vi "demo 0.vi"() -> ()   [LabVIEW 2023]
uses:
  <vilib>/addons/database/Auxilliary.llb/DB Tools Column Info.ctl
  <vilib>/addons/database/Auxilliary.llb/DB Tools DataTypes.ctl
  <vilib>/addons/database/Connection.llb/DB Tools Open Connec (Path).vi
  <vilib>/addons/database/_DB Variant To Data/Database Variant To Data.xnode
  <vilib>/addons/database/NI_Database_API.lvlib
panel:
  in  "?":bool
  out "Attention":string="TYPES YOUR INFORMATIONS "
  in  "connection information 3":path
  in  "column information":T1[](array[typedef])=[{"column name"="stringcol", "data type"=enum."String", "size"=50, "allow null?"=FALSE}, {"column name"="intcol", "data type"=enum."Long (I32)", "size"=0, "allow null?"=TRUE}, {"column name"="doublecol", "data type"=enum."Double (DBL)", "size"=0, "allow null?"=TRUE}]
  in  "LOGING":T3={"PRENOM"="This is a test string", "NOM"="This is a test string", "  TEL"="This is a test string"}
  in  "connection information":path
  out "?":string[][](array[string])
  out "error out":errorcluster
  # "NOM"
  # "TEL"
  # "PRENOM"
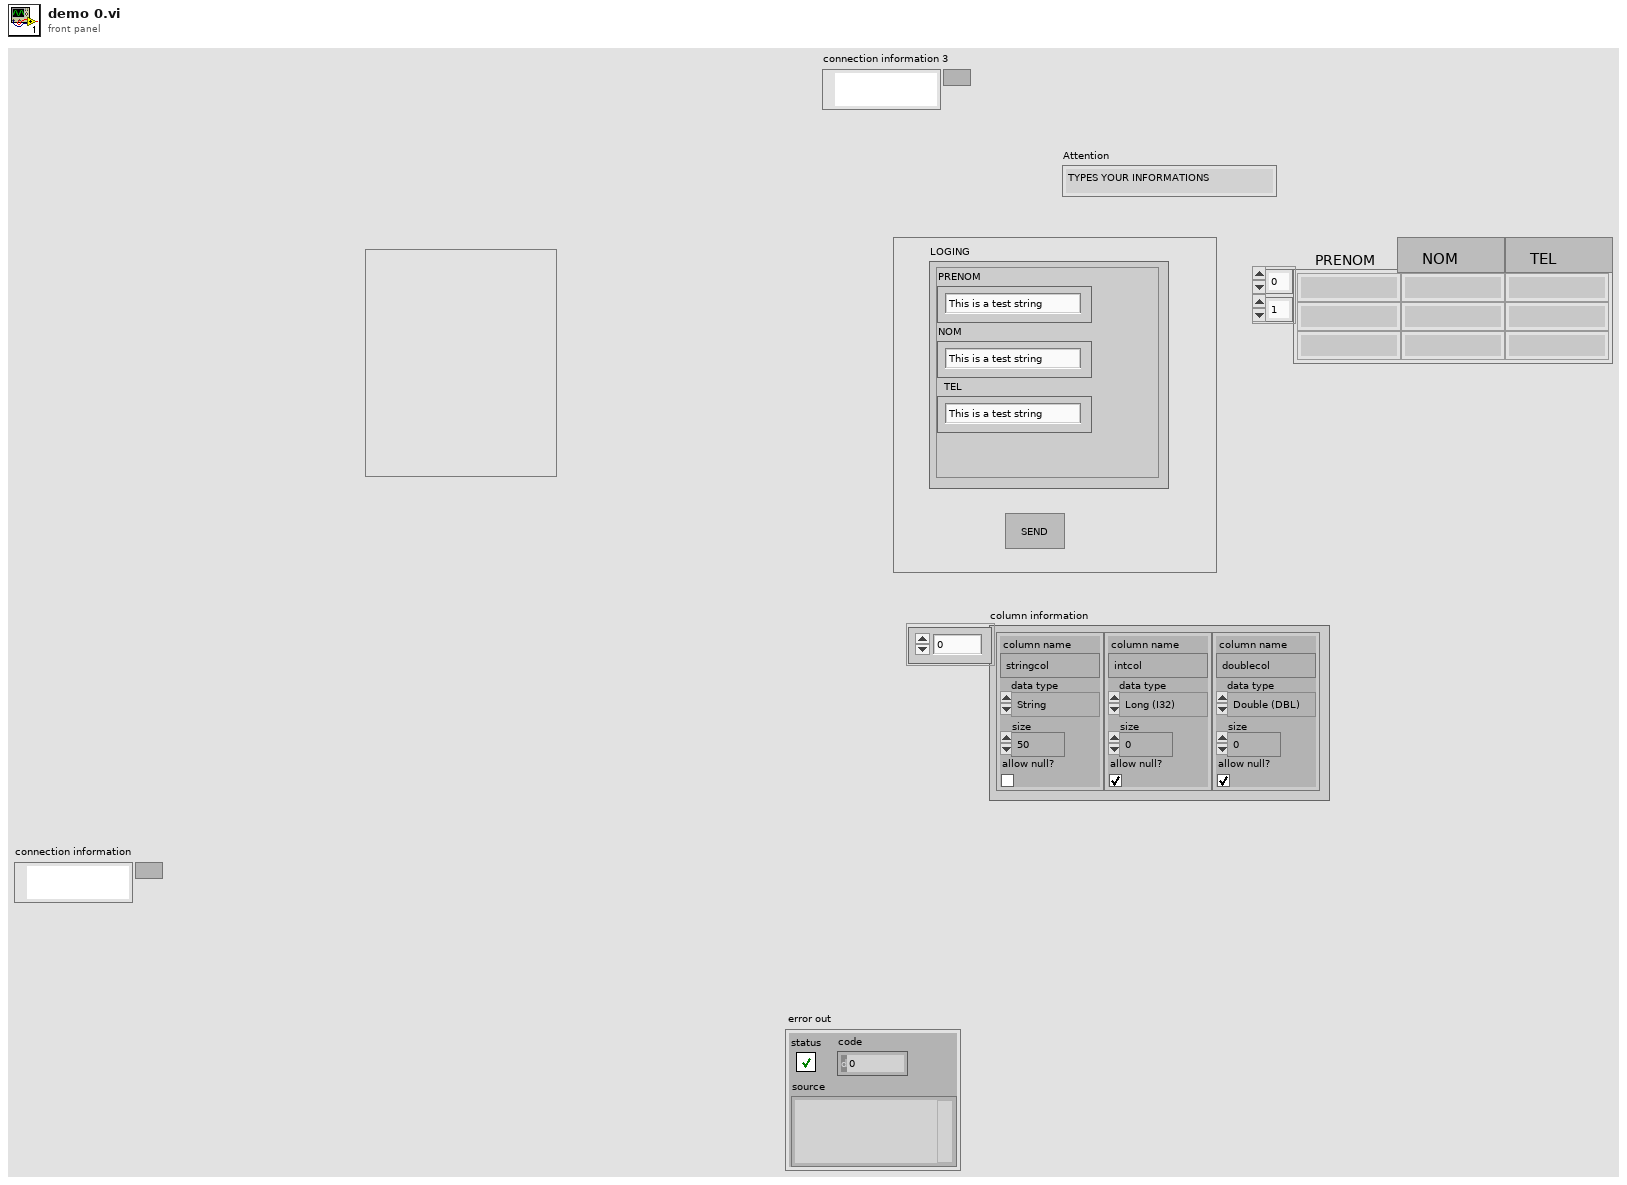
[diagram p1: front panel]
types:
  T1 = typedef "NI_Database_API.lvlib/DB Tools Column Info.ctl" = cluster{"column name":string, "data type":T2, "size":i32, "allow null?":bool}
  T2 = typedef "NI_Database_API.lvlib/DB Tools DataTypes.ctl" = enum16{"String", "Long (I32)", "Single (SGL)", "Double (DBL)", "Date/Time", "Binary"}
  T3 = cluster{"PRENOM":string, "NOM":string, "  TEL":string}
  T4 = typedef "NI_Database_API.lvlib/Conn ObjectReference.ctl" = refnum<k1>
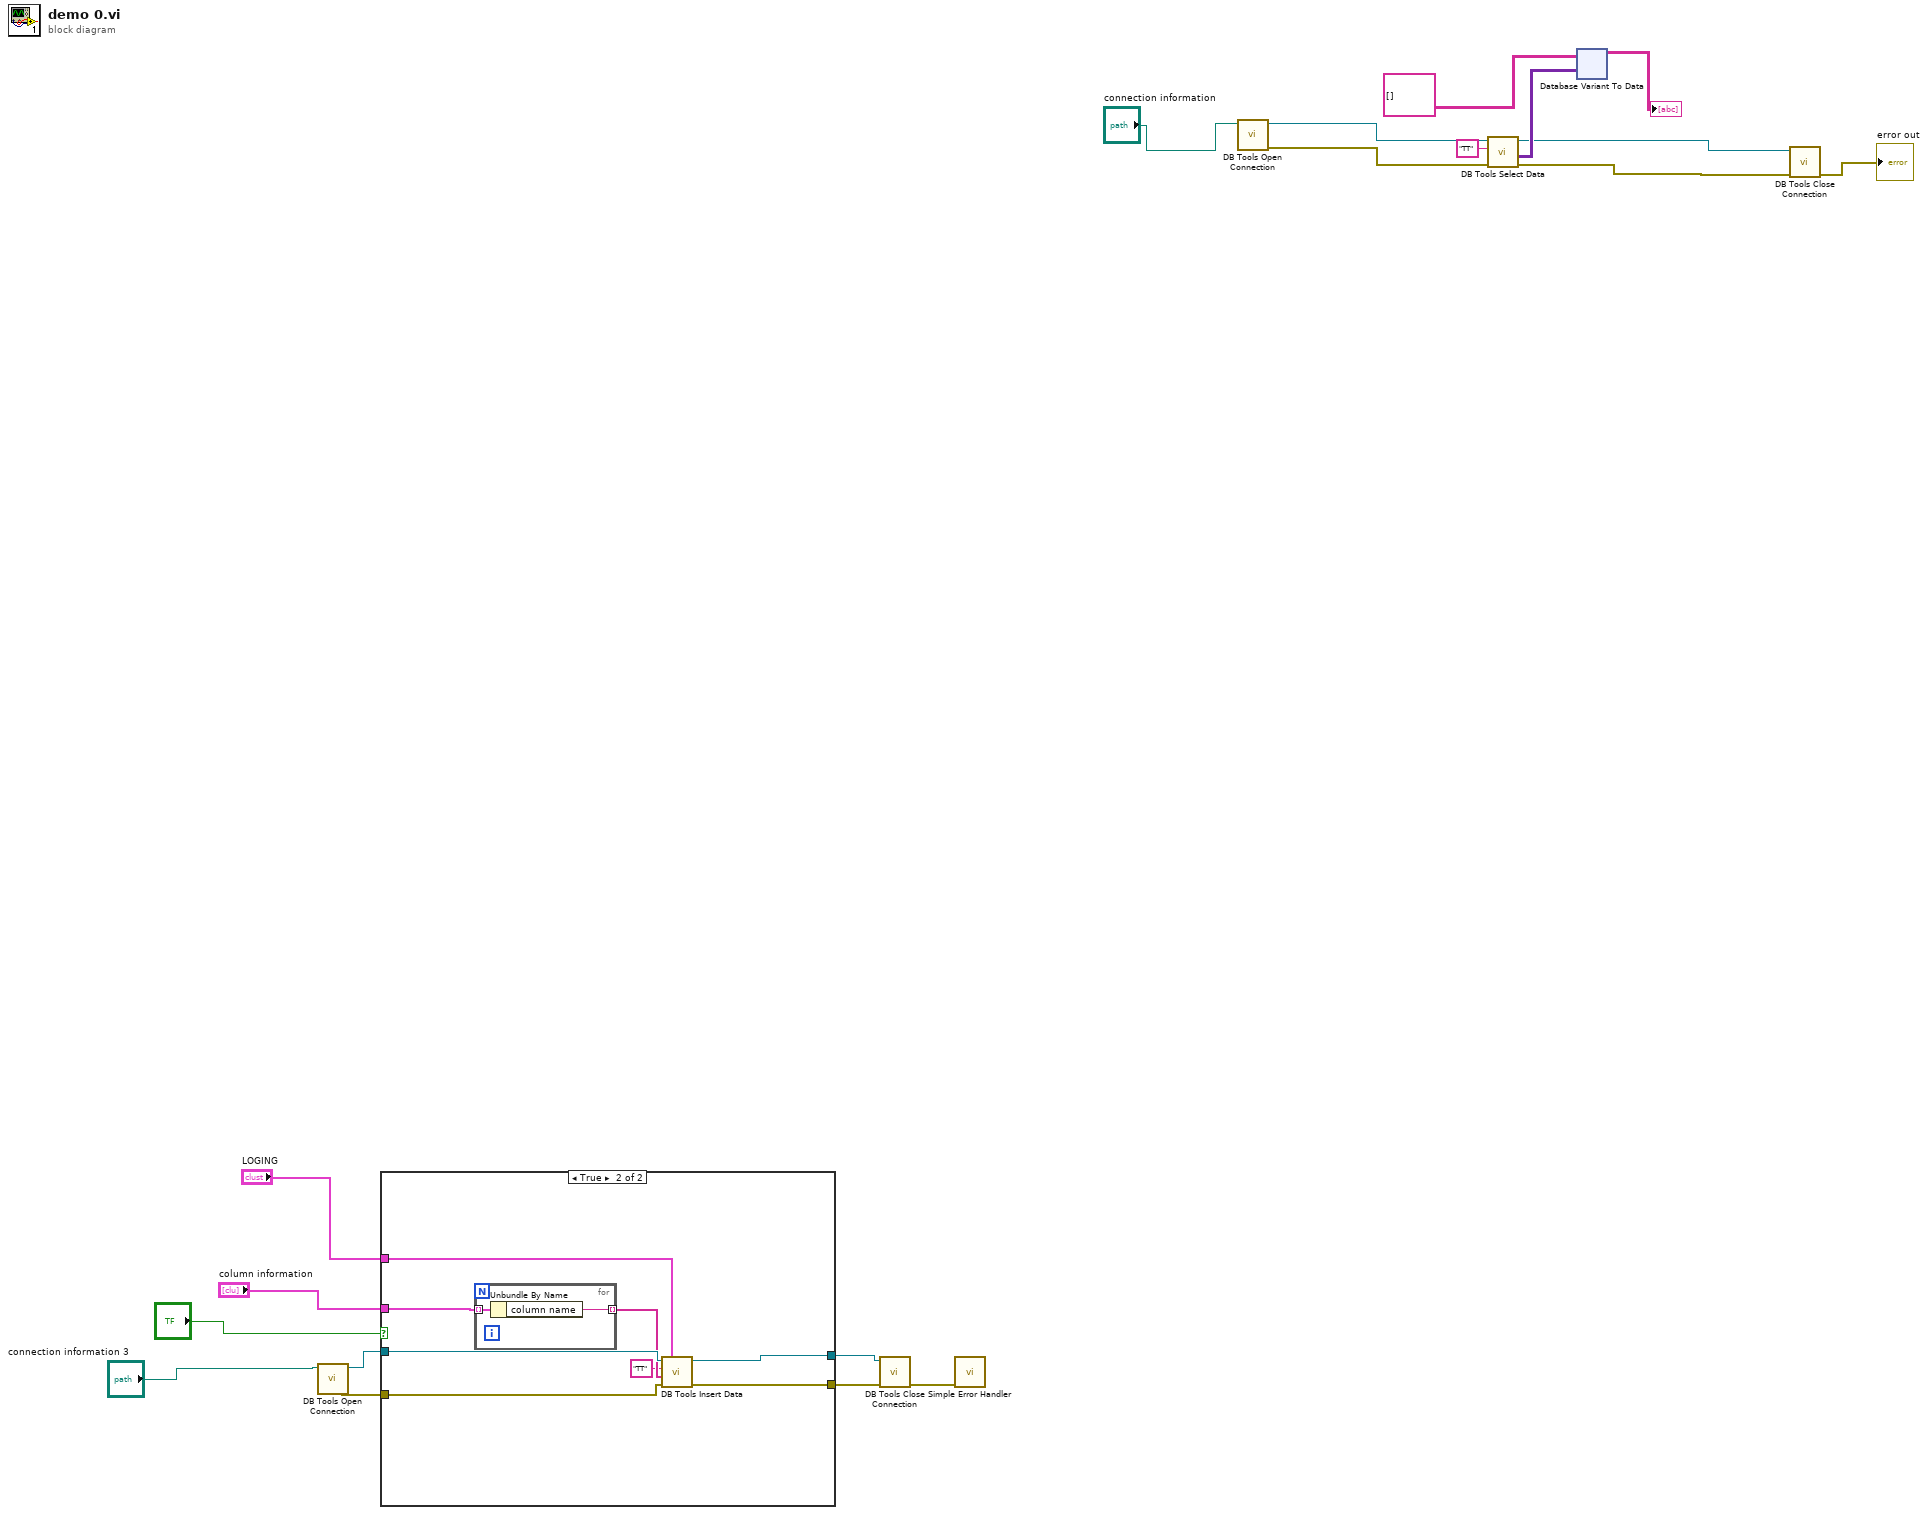
[diagram p0: block diagram]
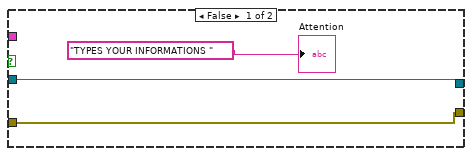
[diagram p2: hidden frame]
diagram:
  n1 = call-poly <vilib>:"DB Tools Open Connection.vi"("connection information"="connection information 3") -> ("error out"=w6:errorcluster, "connection reference"=w9:T4)  [unwired: 7 in]
  n2 = case shown="True" "?" {
    tunnel: w9 -> [w21 w30]
    tunnel: [w21 w29] -> w8
    tunnel: [w20 w28] -> w7
    tunnel: w6 -> [w20 w27]
    tunnel: "LOGING" -> [_ w23]
    tunnel: "column information" -> [_ w26]
    frame False {
      "Attention" <- "TYPES YOUR INFORMATIONS "
    }
    frame True {
      n3 = for {
        tunnel: w26 -> [w32] mode=indexing
        tunnel: [w31] -> w25 mode=indexing
        n4 = Unbundle By Name(w32) -> ("column name"=w31:string)
      }
      n5 = call <vilib>:"DB Tools Insert Data.vi"("data"=w23, "error in (no error)"=w27, "columns"=w25, "table"="TT", "connection reference"=w30) -> ("error out"=w28:errorcluster, "connection reference out"=w29:T4)  [unwired: 5 in]
    }
  }
  n6 = call <vilib>:"DB Tools Close Connection.vi"("error in (no error)"=w7, "connection reference"=w8) -> ("error out"=w11:errorcluster)  [unwired: 5 in]
  n7 = call <vilib>:"Simple Error Handler.vi"("error in (no error)"=w11) -> ()  [unwired: 4 in, 5 out]
  n8 = call-poly <vilib>:"DB Tools Open Connection.vi"("connection information"="connection information") -> ("error out"=w14:errorcluster, "connection reference"=w13:T4)  [unwired: 7 in]
  n9 = call <vilib>:"DB Tools Select Data.vi"("error in (no error)"=w14, "table"="TT", "connection reference"=w13) -> ("error out"=w16:errorcluster, "data"=w15:variant[][], "connection reference out"=w2:T4)  [unwired: 3 in]
  n10 = xnode "Database Variant To Data"("database variant"=w15, "type"=string[][] []) -> ("data"=→"?":string[][])  [unwired: 1 in, 1 out]
  n11 = call <vilib>:"DB Tools Close Connection.vi"("error in (no error)"=w16, "connection reference"=w2) -> ("error out"=→"error out":errorcluster)  [unwired: 5 in]
